vi "Teleop.vi"(10 "Match Info":T1={"Autonomous Elapsed Seconds"=0.0, "TeleOp Elapsed Seconds"=0.0, "Disabled Elapsed Seconds"=0.0, "Visited Autonomous"=FALSE, "Visited TeleOp"=FALSE, "Visited Disabled"=FALSE, "Autonomous Settings"={"Autonomous Style"=enum."Independent", "VI Refnum"=refnum}}, 11 "Call Context":T2) -> ()   [LabVIEW 2016]
doc: "This VI is called for each TeleOp packet received from the DS where the robot is not disabled. It is often used to read from the joysticks and update I/O or to update setpoints for timed control loops. It should complete and return within 20 milliseconds or it may miss DS packets."
uses:
  <vilib>/Rock Robotics/WPI/DriverStation/WPI_DriverStationDerivedRobotMode.ctl
  <vilib>/Rock Robotics/WPI/DriverStation/WPI_DriverStationMatch Info.ctl
  <vilib>/Rock Robotics/WPI/Utilities/WPI_GetSetVariantRefNum.vi
  <vilib>/Rock Robotics/Network Tables/NT Read Boolean.vi
  <vilib>/Rock Robotics/Network Tables/NT Read Number.vi
  <vilib>/Rock Robotics/WPI/Joystick/WPI_JoystickArcadeMapping.vi
panel:
  in  "y":dbl=0.75 format="%#_13g"
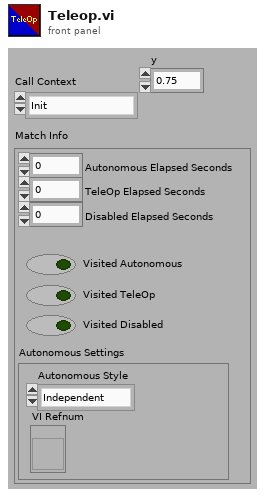
[diagram p1: front panel]
types:
  T1 = typedef "WPI_DriverStationMatch Info.ctl" = cluster{"Autonomous Elapsed Seconds":dbl, "TeleOp Elapsed Seconds":dbl, "Disabled Elapsed Seconds":dbl, "Visited Autonomous":bool, "Visited TeleOp":bool, "Visited Disabled":bool, "Autonomous Settings":cluster{"Autonomous Style":enum16{"Iterative", "Independent"}, "VI Refnum":refnum<vi>}}
  T2 = typedef "WPI_DriverStationDerivedRobotMode.ctl" = enum16{"Init", "Execute", "Stop"}
  T3 = typedef "WPI_JoystickDevRef.ctl" = cluster{"Device":T4}
  T4 = typedef "WPI_JoystickDeviceEnum.ctl" = enum16{"USB 0", "USB 1", "USB 2", "USB 3", "USB 4", "USB 5"}
  T5 = typedef "WPI_MotorControlDeviceRef.ctl" = cluster{"DeviceStatus":errorcluster, "Type":T6, "PWM":cluster{"PWM Channel":T7, "DeadBand":T8}, "CAN":cluster{"Device Number":u8, "SetOutput VI Ref":variant, "GetOutput VI Ref":variant, "Enable VI Ref":variant, "Disable VI Ref":variant, "Data":variant}, "Invert":bool}
  T6 = typedef "WPI_MotorControlType.ctl" = enum16{"PWM", "CAN"}
  T7 = typedef "FPGA_DIOPWMChannel.ctl" = enum8{"PWM 0", "PWM 1", "PWM 2", "PWM 3", "PWM 4", "PWM 5", "PWM 6", "PWM 7", "PWM 8", "PWM 9", "PWM MXP 0", "PWM MXP 1", "PWM MXP 2", "PWM MXP 3", "PWM MXP 4", "PWM MXP 5", "PWM MXP 6", "PWM MXP 7", "PWM MXP 8", "PWM MXP 9", "Invalid"}
  T8 = typedef "WPI_PWMDeadband.ctl" = cluster{"Name":string, "maxPositivePwm":i32, "minPositivePwm":i32, "centerPwm":i32, "maxNegativePwm":i32, "minNegativePwm":i32, "angularRange":u16}
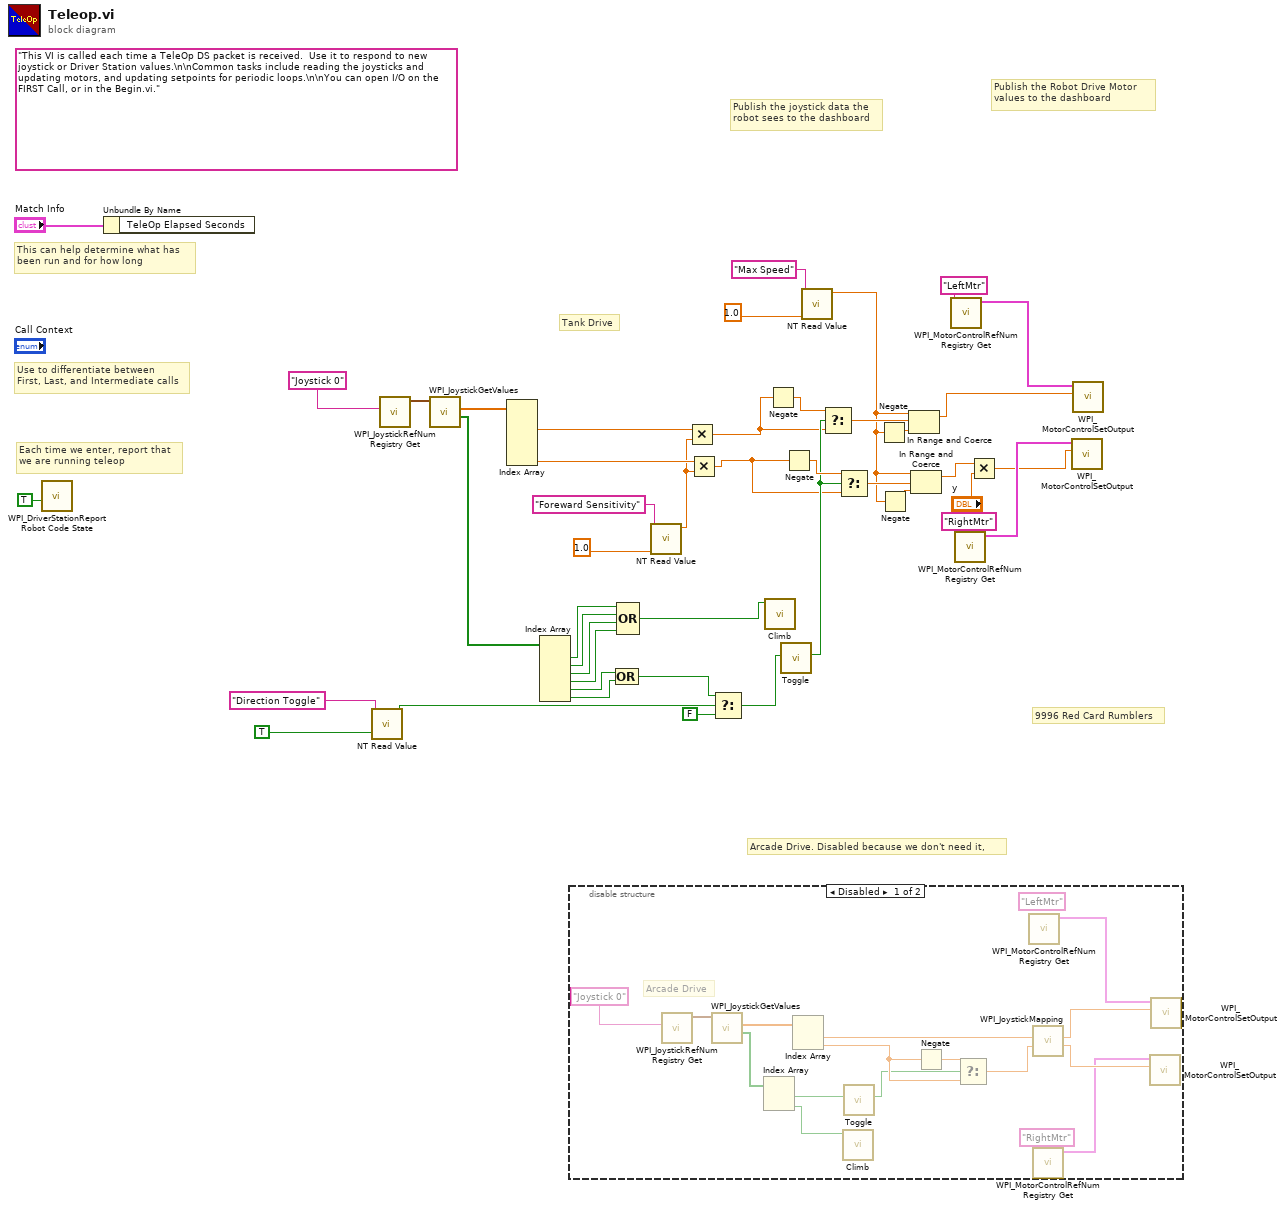
[diagram p0: block diagram]
diagram:
  (unwired) "This VI is called each time a TeleOp DS packet is received.  Use it to respond to new joystick or Driver Station values.\n\nCommon tasks include reading the joysticks and updating motors, and updating setpoints for periodic loops.\n\nYou can open I/O on the FIRST Call, or in the Begin.vi."
  # "9996 Red Card Rumblers"
  # "Arcade Drive. Disabled because we don't need it,"
  # "Tank Drive"
  # "Publish the Robot Drive Motor\nvalues to the dashboard"
  # "Publish the joystick data the\nrobot sees to the dashboard"
  # "Each time we enter, report that\nwe are running teleop"
  # "Use to differentiate between\nFirst, Last, and Intermediate calls"
  # "This can help determine what has\nbeen run and for how long"
  n1 = call <vilib>:"WPI_DriverStationReport Robot Code State.vi"("TeleOp"=TRUE ("Autonomous")) -> ()  [unwired: 10 in, 1 out]
  n2 = Unbundle By Name("Match Info") -> ()  [unwired: 1 out]
  n3 = call-poly <vilib>:"NT Read Value.vi"("Default Value"=TRUE, "Name"="Direction Toggle") -> ("Boolean"=w21:bool)  [unwired: 8 in, 1 out]
  n4 = call <vilib>:"WPI_JoystickRefNum Registry Get.vi"("refnum name"="Joystick 0") -> ("JoystickDevRef"=w38:T3)  [unwired: 1 in, 9 out]
  n5 = call <vilib>:"WPI_JoystickGetValues.vi"("JoystickDevRef"=w38) -> ("Buttons"=w40:bool[], "Axes"=w39:dbl[])  [unwired: 6 in, 3 out]
  n6 = Index Array(array=w39) -> (element #2=w16:dbl, element #6=w17:dbl)  [unwired: 6 in, 4 out]
  n7 = Index Array(array=w40) -> (element #1=w26:bool, element #2=w27:bool, element #3=w28:bool, element #4=w29:bool, element #5=w31:bool, element #6=w30:bool)  [unwired: 6 in]
  n8 = disable-structure shown="Disabled" {
    frame Disabled {
      (unwired) "LeftMtr" ("refnum name")
      # "Arcade Drive"
      n9 = call <vilib>:"WPI_JoystickRefNum Registry Get.vi"("refnum name"="Joystick 0") -> ("JoystickDevRef"=w46:T3)  [unwired: 1 in, 9 out]
      n10 = call <vilib>:"WPI_JoystickGetValues.vi"("JoystickDevRef"=w46) -> ("Buttons"=w48:bool[], "Axes"=w47:dbl[])  [unwired: 6 in, 3 out]
      n11 = Index Array(array=w48) -> (element #1=w55:bool, element #2=w60:bool)  [unwired: 2 in]
      n12 = Index Array(array=w47) -> (element #1=w54:dbl, element #2=w58:dbl)  [unwired: 2 in]
      n13 = call "Climb.vi"("Climb"=w60) -> ()  [unwired: 11 in]
      n14 = call "Toggle.vi"("Input"=w55) -> ("Output"=w56:bool)  [unwired: 10 in]
      n15 = Negate(x=w58) -> (-x=w57:dbl)
      n16 = Select(t=w57, s=w56, f=w58) -> (s? t:f=w59:dbl)
      n17 = call <vilib>:"WPI_MotorControlRefNum Registry Get.vi"() -> ("MotorControlDevRef"=w49:T5)  [unwired: 10 in, 1 out]
      n18 = call-poly <vilib>:"WPI_JoystickMapping.vi"("Y axis value"=w59, "X axis value"=w54) -> ("Right Motor Value"=w53:dbl, "Left Motor Value"=w52:dbl)  [unwired: 8 in]
      n19 = call <vilib>:"WPI_MotorControlRefNum Registry Get.vi"("refnum name"="RightMtr") -> ("MotorControlDevRef"=w50:T5)  [unwired: 9 in, 1 out]
      n20 = call <vilib>:"WPI_MotorControlSetOutput.vi"("Output"=w53, "MotorControlDevRef"=w50) -> ()  [unwired: 7 in, 3 out]
      n21 = call <vilib>:"WPI_MotorControlSetOutput.vi"("Output"=w52, "MotorControlDevRef"=w49) -> ()  [unwired: 7 in, 3 out]
    }
    frame Enabled {
    }
  }
  n22 = Compound Arithmetic op=OR(w31, w30) -> (w22:bool)
  n23 = Compound Arithmetic op=OR(w26, w27, w28, w29) -> (w25:bool)
  n24 = call-poly <vilib>:"NT Read Value.vi"("Default Value"=1.0, "Name"="Foreward Sensitivity") -> ("Numeric"=w13:dbl)  [unwired: 8 in, 1 out]
  n25 = Multiply(x=w16, y=w13) -> (x*y=w15:dbl)
  n26 = Multiply(x=w17, y=w13) -> (x*y=w12:dbl)
  n27 = Select(t=w22, s=w21, f=FALSE) -> (s? t:f=w19:bool)
  n28 = call "Climb.vi"("Climb"=w25) -> ()  [unwired: 11 in]
  n29 = Negate(x=w15) -> (-x=w34:dbl)
  n30 = call "Toggle.vi"("Input"=w19) -> ("Output"=w32:bool)  [unwired: 10 in]
  n31 = Negate(x=w12) -> (-x=w33:dbl)
  n32 = call-poly <vilib>:"NT Read Value.vi"("Default Value"=1.0, "Name"="Max Speed") -> ("Numeric"=w5:dbl)  [unwired: 8 in, 1 out]
  n33 = Select(t=w34, s=w32, f=w15) -> (s? t:f=w11:dbl)
  n34 = Select(t=w33, s=w32, f=w12) -> (s? t:f=w8:dbl)
  n35 = Negate(x=w5) -> (-x=w7:dbl)
  n36 = Negate(x=w5) -> (-x=w6:dbl)
  n37 = In Range and Coerce(upper limit=w5, x=w11, lower limit=w7) -> (coerced(x)=w4:dbl)  [unwired: 1 out]
  n38 = In Range and Coerce(upper limit=w5, x=w8, lower limit=w6) -> (coerced(x)=w2:dbl)  [unwired: 1 out]
  n39 = call <vilib>:"WPI_MotorControlRefNum Registry Get.vi"("refnum name"="LeftMtr") -> ("MotorControlDevRef"=w41:T5)  [unwired: 9 in, 1 out]
  n40 = call <vilib>:"WPI_MotorControlRefNum Registry Get.vi"("refnum name"="RightMtr") -> ("MotorControlDevRef"=w42:T5)  [unwired: 9 in, 1 out]
  n41 = Multiply(x=w2, y="y") -> (x*y=w3:dbl)
  n42 = call <vilib>:"WPI_MotorControlSetOutput.vi"("Output"=w3, "MotorControlDevRef"=w42) -> ()  [unwired: 7 in, 3 out]
  n43 = call <vilib>:"WPI_MotorControlSetOutput.vi"("Output"=w4, "MotorControlDevRef"=w41) -> ()  [unwired: 7 in, 3 out]
